vi "Launch Message Handler.vi"(8 "error in (no error)":errorcluster, 11 "Consumer":refnum<class "Abstract Consumer.lvclass">) -> (0 "error out":errorcluster)   [LabVIEW 2024, in "AIM ARINC 429 Engine.lvlib" / "Implementation.lvlib" / "Word Logging.lvlib"]
uses:
  Word Logging.lvlib
  <vilib>/NI/VeriStand Custom Device Messaging/Consumer/Abstract Consumer/Abstract Consumer.lvclass
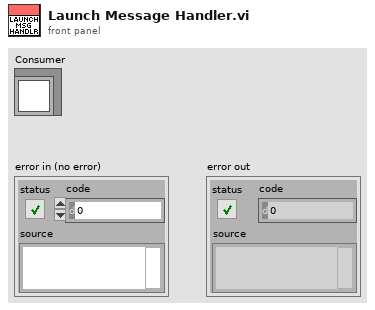
[diagram p1: front panel]
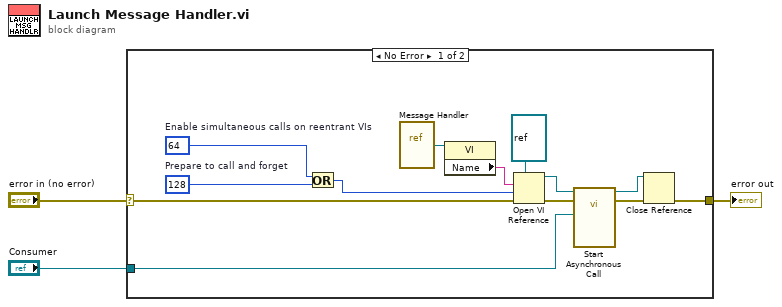
[diagram p0: block diagram]
diagram:
  n1 = case shown="No Error" "error in (no error)" {
    selector: "error in (no error)" -> [w16 w17]
    tunnel: [w5 w17] -> w2
    tunnel: "Consumer" -> [w6 _]
    frame No Error {
      w11 = 64  # Enable simultaneous calls on reentrant VIs
      w12 = 128  # Prepare to call and forget
      n2 = Or(x=w11, y=w12) -> (x .or. y?=w10:i32)
      n3 = vi-ref "Message Handler.vi"() -> (w9:refnum<vi>)
      n4 = property class="VI"(reference=w9) -> ("Name"=w7:string)  [unwired: 1 in, 2 out]
      n5 = Open VI Reference(type specifier VI Refnum (for type only)=refnum<vi> refnum, vi path=w7, options=w10, error in (no error)=w16) -> (vi reference=w15:refnum<vi>, error out=w14:errorcluster)  [unwired: 2 in]
      n6 = call-by-ref "Start Asynchronous Call"(reference=w15, error in=w14, "Consumer"=w6) -> (reference out=w4:refnum<vi>, error out=w13:errorcluster)  [unwired: 11 in]
      n7 = Close Reference(reference=w4, error in (no error)=w13) -> (error out=w5:errorcluster)
    }
    frame Error {
    }
  }
  "error out" <- w2
